vi "Configure Trigger Event SMU End Pulse.vi"(0 "VISA resource name":refnum<visa-resource-name>, 5 "Source Measure Unit Channel (0: Channel A)":i32(ring) items=["Channel A", "Channel B"], 7 "Event ID":string, 11 "error in (no error)":errorcluster) -> (4 "VISA resource name out":refnum<visa-resource-name>, 15 "error out":errorcluster)   [LabVIEW 2017, in "Keithley 2600 Series.lvlib"]
doc: "Configures the event that will cause the end pulse event detector to enter the detected state."
uses:
  <instrlib>/Keithley 2600 Series/Keithley 2600 Series.lvlib
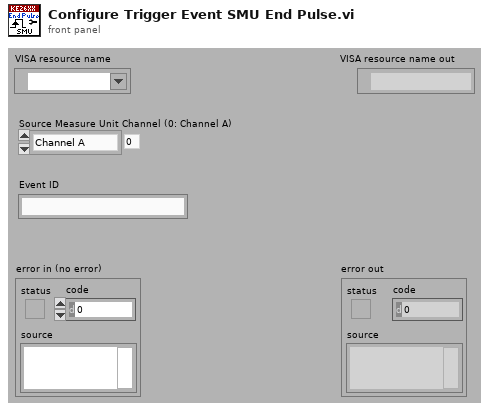
[diagram p1: front panel]
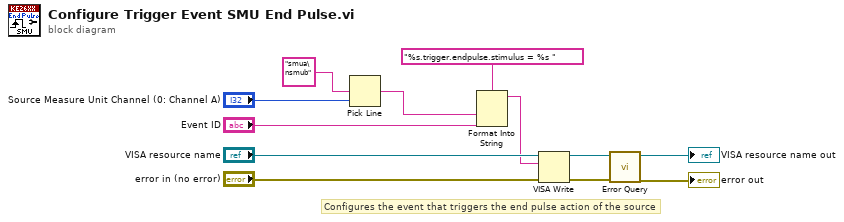
[diagram p0: block diagram]
diagram:
  # "Configures the event that triggers the end pulse action of the source"
  n1 = Pick Line(multi-line string="smua\nsmub", line index="Source Measure Unit Channel (0: Channel A)") -> (output string=w1:string)  [unwired: 1 in]
  n2 = Format Into String(format string="%s.trigger.endpulse.stimulus = %s ", w1, "Event ID") -> (resulting string=w2:string)  [unwired: 2 in, 1 out]
  n3 = VISA Write(VISA resource name="VISA resource name", write buffer=w2, error in (no error)="error in (no error)") -> (VISA resource name out=w8:refnum<visa-resource-name>, error out=w7:errorcluster)  [unwired: 1 out]
  n4 = call <instrlib>:"Error Query.vi"("error in (no error)"=w7, "VISA resource name"=w8) -> ("error out"=→"error out":errorcluster, "VISA resource name out"=→"VISA resource name out":refnum<visa-resource-name>)  [unwired: 6 in, 2 out]
